vi "RT - Listener.vi"() -> ()   [LabVIEW 2017]
panel:
  out "Number Received from Host":i32
  in  "stop":bool
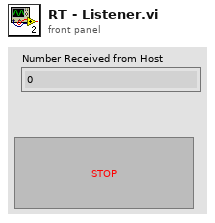
[diagram p1: front panel]
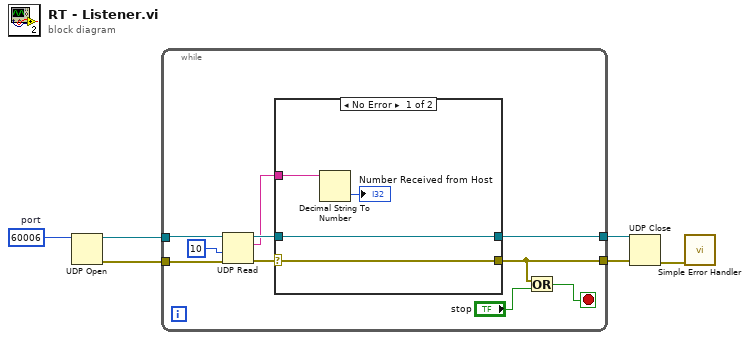
[diagram p0: block diagram]
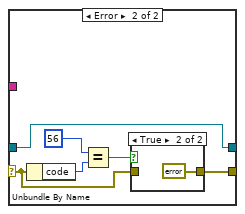
[diagram p2: hidden frame]
diagram:
  w4 = u16 60006  # port
  n1 = UDP Open(11:w4) -> (port=w6:refnum<k16>, 0:w5:errorcluster)  [unwired: 4 in, 1 out]
  n2 = while {
    tunnel: w6 -> [w16]
    tunnel: w5 -> [w15]
    tunnel: [w9] -> w2
    tunnel: [w8] -> w1
    stop <- w12 stop-if-true
    n3 = UDP Read(connection ID=w16, timeout ms (25000)=10, 8:w15) -> (data out=w7:string, error out=w10:errorcluster, 3:w11:refnum<k16>)  [unwired: 1 in, 2 out]
    n4 = case shown="No Error" w10 {
      selector: w10 -> [w20 w22]
      tunnel: w11 -> [w19 w21]
      tunnel: w7 -> [w18 _]
      tunnel: [w20 w23] -> w8
      tunnel: [w19 w21] -> w9
      frame No Error {
        n5 = Decimal String To Number(string=w18) -> (number=→"Number Received from Host":i32)  [unwired: 2 in, 1 out]
      }
      frame Error {
        n6 = Unbundle By Name(w22) -> ("code"=w26:i32)
        n7 = Equal?(x=56, y=w26) -> (x = y?=w24:bool)
        n8 = case shown="True" w24 {
          tunnel: [w27 errorcluster {"status"=FALSE, "code"=0, "source"=""} ("error constant")] -> w23
          tunnel: w22 -> [w27 _]
          frame False {
          }
          frame True {
          }
        }
      }
    }
    n9 = Or(x=w8, y="stop") -> (x .or. y?=w12:bool)
  }
  n10 = UDP Close(connection ID=w2, 8:w1) -> (error out=w3:errorcluster)  [unwired: 1 out]
  n11 = call <vilib>:"Simple Error Handler.vi"("error in (no error)"=w3) -> ()  [unwired: 4 in, 5 out]
